vi "TaskMon_GetProcessesAndIDs.vi"(8 "error in (no error)":errorcluster) -> (0 "error out":errorcluster, 3 "ProcesesList":string[](array[string]), 4 "return":i32, 5 "IDs":u32[](array[numeric]))   [LabVIEW 2020]
uses:
  processHandles.dll
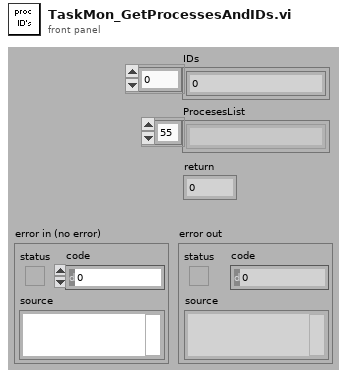
[diagram p1: front panel]
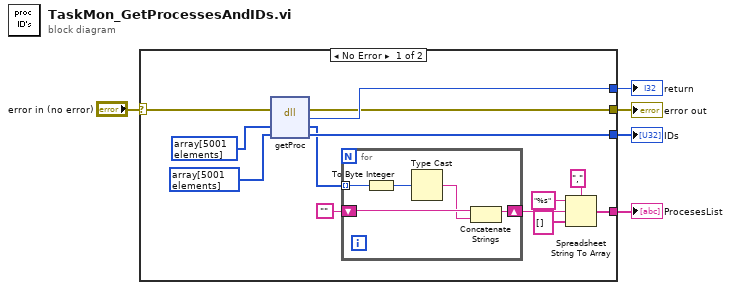
[diagram p0: block diagram]
diagram:
  n1 = case shown="No Error" "error in (no error)" {
    selector: "error in (no error)" -> [w6 w24]
    tunnel: [w18 _] -> w5
    tunnel: [w16 _] -> w4
    tunnel: [w10 _] -> w3
    tunnel: [w7 w24] -> w2
    frame No Error {
      n2 = dll-call lib="E:/LabVIEW 2020 Toolkits/toolkits_lv2020_32bit/TaskManager/processHandles.dll" fn="getProc"(error in=w6, "procs"=u16[] array[5001 elements] ("procs 3"), "IDs"=u32[] array[5001 elements]) -> (error out=w7:errorcluster, "return type"=w18:i32, "procs"=w14:u16[], "IDs"=w16:u32[])  [unwired: 2 in, 1 out]
      n3 = for {
        tunnel: w14 -> [w21] mode=indexing
        shift-right: [w22] -> w13
        shift-left: "" -> [w23]
        n4 = To Byte Integer(number=w21) -> (8bit integer=w20:i8)
        n5 = Type Cast(x=w20) -> (*(type *) &x=w19:string)  [unwired: 1 out]
        n6 = Concatenate Strings(w23, w19) -> (w22:string)
      }
      n7 = Spreadsheet String To Array(delimiter (Tab)=",", format string="%s", spreadsheet string=w13, array type (2D Dbl)=string[] []) -> (array=w10:string[])
    }
    frame Error {
    }
  }
  "return" <- w5
  "IDs" <- w4
  "ProcesesList" <- w3
  "error out" <- w2
